vi "Handle Error.vi"(8 "error in (no error)":errorcluster, 11 "DAQ Actor in":refnum<class "DAQ Actor.lvclass">) -> (0 "error out":errorcluster, 2 "stop actor?":bool=TRUE, 3 "DAQ Actor out":refnum<class "DAQ Actor.lvclass">)   [LabVIEW 2018, in "Data Acquisition.lvlib" / "DAQ Actor.lvclass"]
doc: "(<B>Filename</B>: Actor Framework.lvlib:Actor.lvclass:Handle Error.vi)\n\nDefines how the actor handles an error that occurred while processing a message.\n\nBy default, this method does nothing except stop the actor. This method also treats error code 43 (coming from <B>error in</B>) as a sign that the actor shut down normally. In this situation, the Handle Error method does not return the error on <B>error out</B>, meaning the actor's caller will not receive it. All other error codes will be returned on <B>error out</B>.\n\nA descendant class may override this method to change this behavior."
uses:
  DAQ Actor.lvclass
  C:/Program Files (x86)/National Instruments/LabVIEW 2018/vi.lib/ActorFramework/Actor/Actor.lvclass
  <vilib>/ActorFramework/Actor/Actor.lvclass/Actor.ctl
  <vilib>/ActorFramework/Message Enqueuer/Message Enqueuer.lvclass/Message Enqueuer.ctl
  Cfg Grandmaster/Cfg Grandmaster Messages/Update Runtime Error Indicator Msg/Update Runtime Error Indicator Msg.lvclass/Update Runtime Error Indicator Msg.ctl
  <vilib>/ActorFramework/Message Enqueuer/Enqueue.vi
  Cfg Grandmaster/DAQMan Messages/Stop All DAQ Msg/Stop All DAQ Msg.lvclass
  C:/Program Files (x86)/National Instruments/LabVIEW 2018/vi.lib/ActorFramework/Message/Message.lvclass
  Cfg Grandmaster/Cfg Grandmaster Messages/Update Runtime Error Indicator Msg/Update Runtime Error Indicator Msg.lvclass
  <vilib>/ActorFramework/Message Priority Queue/Priority Enqueue.vi
  <vilib>/ActorFramework/Actor/Actor.lvclass
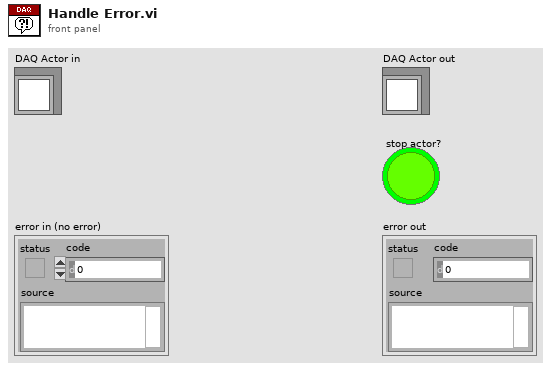
[diagram p1: front panel]
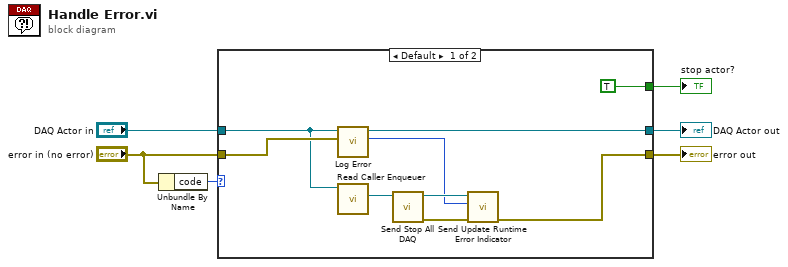
[diagram p0: block diagram]
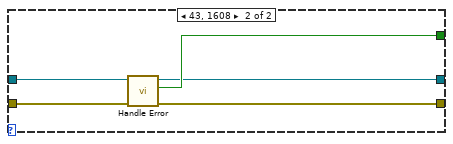
[diagram p2: hidden frame]
diagram:
  n1 = Unbundle By Name("error in (no error)") -> ("code"=w2:i32)
  n2 = case shown="Default" w2 {
    tunnel: [w7 w20] -> w6
    tunnel: [TRUE ("stop actor?") w19] -> w5
    tunnel: [w14 w18] -> w4
    tunnel: "error in (no error)" -> [w13 w17]
    tunnel: "DAQ Actor in" -> [w12 w16]
    frame Default {
      n3 = call "Log Error.vi"("error in (no error)"=w13, "DAQ Actor in"=w12) -> ("Error Count"=w9:u32, "DAQ Actor out"=w14:refnum<class "DAQ Actor.lvclass">)  [unwired: 7 in, 1 out]
      n4 = call <vilib>:"Read Caller Enqueuer.vi"("Actor"=w12) -> ("Caller Enqueuer"=w11:refnum<class "Message Enqueuer.lvclass">)  [unwired: 10 in]
      n5 = call "Send Stop All DAQ.vi"("Message Enqueuer"=w11) -> ("error out"=w8:errorcluster, "Message Enqueuer out"=w10:refnum<class "Message Enqueuer.lvclass">)  [unwired: 9 in]
      n6 = call "Send Update Runtime Error Indicator.vi"("error in (no error)"=w8, "Error Count"=w9, "Message Enqueuer"=w10) -> ("error out"=w7:errorcluster)  [unwired: 7 in, 1 out]
    }
    frame 43, 1608 {
      n7 = call-parent "Handle Error.vi"("error in (no error)"=w17, "Actor in"=w16) -> ("error out"=w20:errorcluster, "stop actor?"=w19:bool, "Actor out"=w18:refnum<class "DAQ Actor.lvclass">)  [unwired: 7 in]
    }
  }
  "DAQ Actor out" <- w4
  "error out" <- w6
  "stop actor?" <- w5
